vi "Create Sysdef Channels from DMAs Configuration.vi"(6 "Use NI-VS":bool, 8 "error in (no error)":errorcluster, 10 "Device Ref":T1=18446744073709551615 format="%.0x", 11 "DMAs":T2[](array[typedef])) -> (0 "error out":errorcluster, 3 "Device Ref Out":T1=18446744073709551615 format="%.0x")   [LabVIEW 2019, in "RefMem DMA System Explorer.lvlib"]
uses:
  controls/Typedef_DMA Instance.ctl
  controls/Typedef_DMA Block Settings.ctl
  controls/Data Channel Type.ctl
  controls/Typedef_Channel Settings.ctl
  <vilib>/NI VeriStand/Custom Device API/Custom Device Item Ref.ctl
  <vilib>/NI VeriStand/Custom Device API/Custom Device Channel.ctl
  <vilib>/NI VeriStand/Custom Device API/Custom Device Channel Type.ctl
  Shared/Constants.vi
  <vilib>/NI VeriStand/Custom Device API/Set Item Property (U16).vi
  <vilib>/NI VeriStand/Custom Device API/Set Item Property (U32).vi
  RefMem DMA System Explorer.lvlib
  <vilib>/NI VeriStand/Custom Device API/Custom Device API.lvlib
  Shared/RefMem DMA Shared.lvlib
panel:
  out "Creation Progress":u32(slide) scale=0.0..100.0
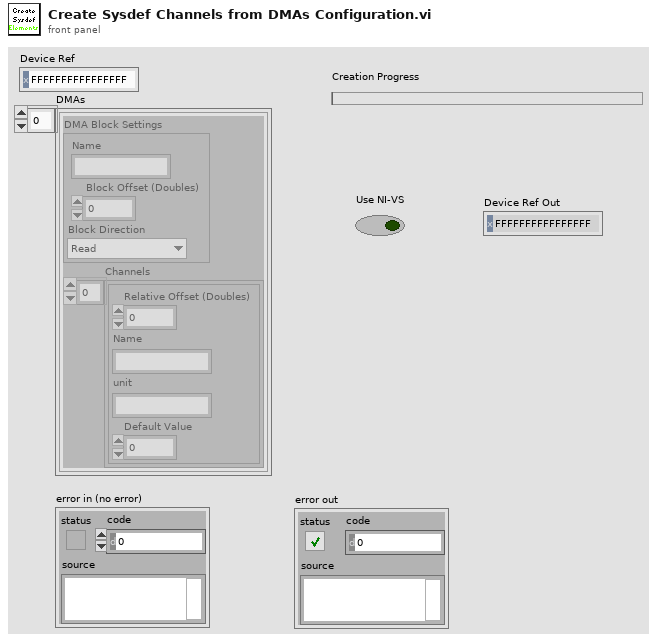
[diagram p1: front panel]
types:
  T1 = typedef "Custom Device API.lvlib/Custom Device Item Ref.ctl" = u64
  T2 = typedef "RefMem DMA System Explorer.lvlib/Typedef_DMA Instance.ctl" = cluster{"DMA Block Settings":T3, "Channels":T5[]}
  T3 = typedef "RefMem DMA System Explorer.lvlib/Typedef_DMA Block Settings.ctl" = cluster{"Name":string, " Block Offset (Doubles)":u32, "Block Direction":T4}
  T4 = typedef "RefMem DMA System Explorer.lvlib/Data Channel Type.ctl" = enum16{"Read", "Write"}
  T5 = typedef "RefMem DMA System Explorer.lvlib/Typedef_Channel Settings.ctl" = cluster{"Relative Offset (Doubles)":u32, "Name":string, "unit":string, "Default Value":dbl}
  T6 = typedef "Custom Device API.lvlib/Custom Device Channel.ctl" = cluster{"Type":T7, "Units":string, "Default Value":dbl, "Faultable":bool, "Scalable":bool}
  T7 = typedef "Custom Device API.lvlib/Custom Device Channel Type.ctl" = enum16{"Input", "Output"}
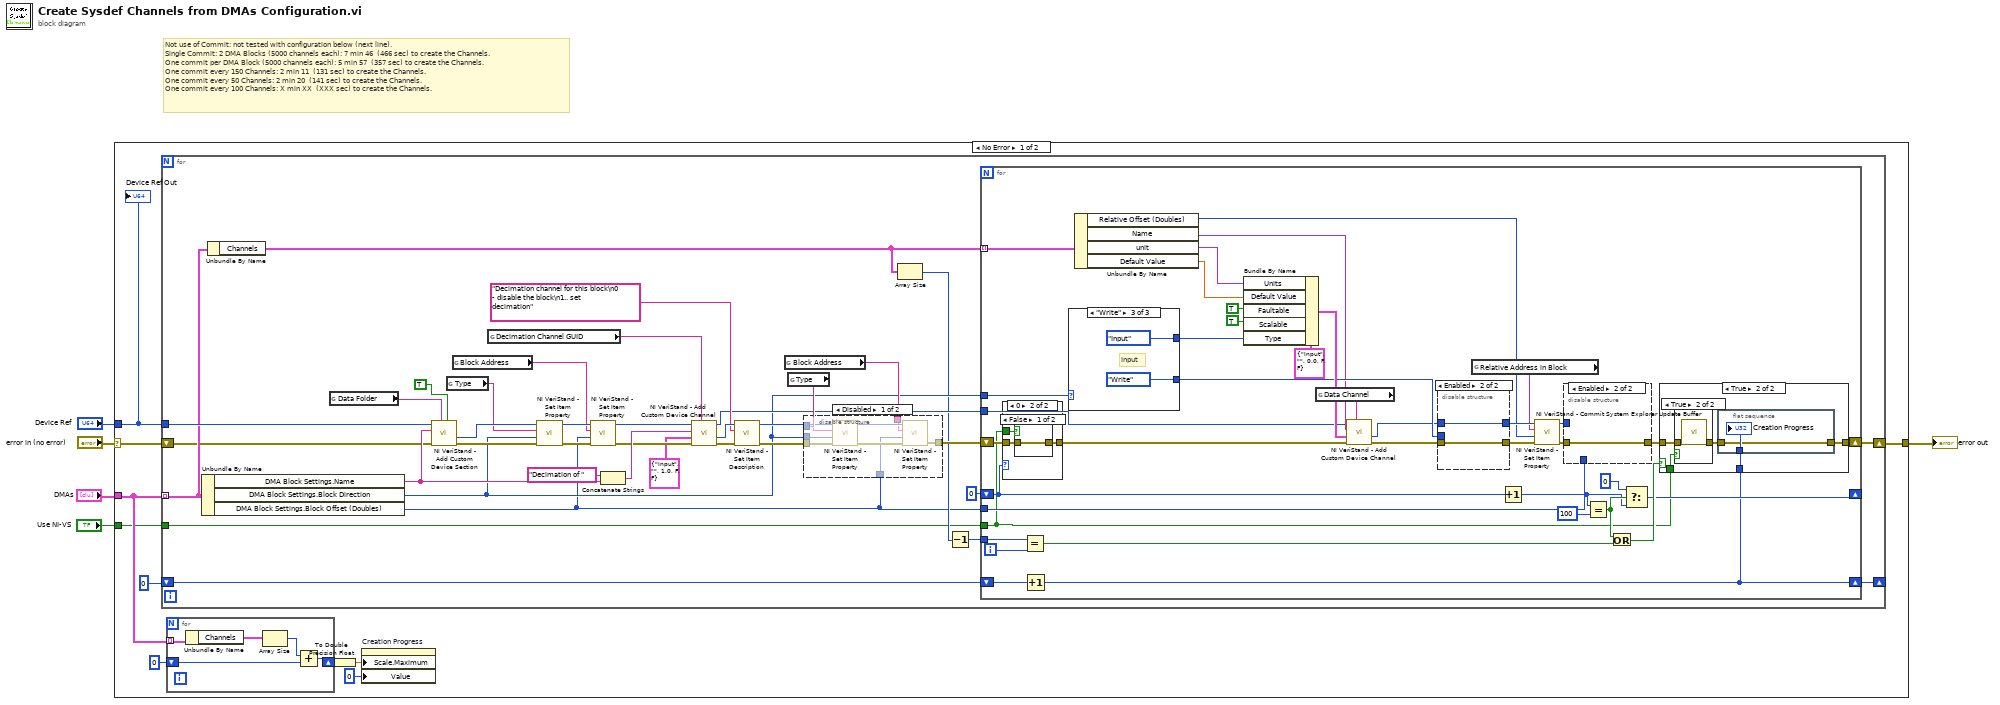
[diagram p0: block diagram]
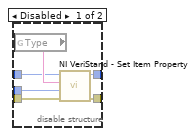
[diagram p3: hidden frame]
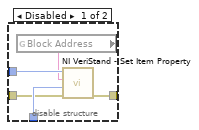
[diagram p4: hidden frame]
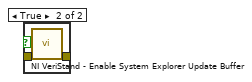
[diagram p6: hidden frame]
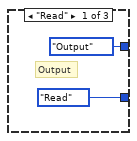
[diagram p9: hidden frame]
diagram:
  # "Not use of Commit: not tested with configuration below (next line).\nSingle Commit: 2 DMA Blocks (5000 channels each): 7 min 46  (466 sec) to create the Channels.\nOne commit per DMA Block (5000 channels each): 5 min 57  (357 sec) to create the Channels.\nOne commit every 150 Channels: 2 min 11  (131 sec) to create the Channels.\nOne commit every 50 Channels: 2 min 20  (141 sec) to create the Channels.\nOne commit every 100 Channels: X min XX  (XXX sec) to create the Channels."
  n1 = case shown="No Error" "error in (no error)" {
    selector: "error in (no error)" -> [w7 w143]
    tunnel: "Device Ref" -> [w15 _]
    tunnel: [w14 w143] -> w4
    tunnel: "DMAs" -> [w13 _]
    tunnel: "Use NI-VS" -> [w6 _]
    frame No Error {
      n2 = for {
        shift-right: [w29] -> w14
        shift-left: w7 -> [w30]
        tunnel: w15 -> [w36]
        tunnel: w13 -> [w34] mode=indexing
        shift-right: [w23] -> _
        shift-left: u32 0 -> [w24]
        tunnel: w6 -> [w21]
        n3 = Unbundle By Name(w34) -> ("DMA Block Settings.Name"=w37:string, "DMA Block Settings.Block Direction"=w31:T4, "DMA Block Settings.Block Offset (Doubles)"=w22:u32)
        n4 = Unbundle By Name(w34) -> ("Channels"=w28:T5[])
        n5 = global read "Constants.vi" "Data Folder"() -> (w42:string)
        n6 = call <vilib>:"NI VeriStand - Add Custom Device Section.vi"("Highlight? (F)"=TRUE, "GUID (Default Section)"=w42, "error in (no error)"=w30, "Section Name"=w37, "Parent Ref in"=w36) -> ("error out"=w45:errorcluster, "Section Ptr"=w49:T1)  [unwired: 3 in, 2 out]
        n7 = global read "Constants.vi" "Type"() -> (w44:string)
        n8 = global read "Constants.vi" "Block Address"() -> (w43:string)
        n9 = global read "Constants.vi" "Decimation Channel GUID"() -> (w52:string)
        n10 = call-poly <vilib>:"NI VeriStand - Set Item Property.vi"("error in (no error)"=w45, "Value"=w31, "Property Name"=w44, "Item Ref in"=w49) -> ("error out"=w46:errorcluster, "Item Ref out"=w47:T1)  [unwired: 5 in, 1 out]
        n11 = call-poly <vilib>:"NI VeriStand - Set Item Property.vi"("error in (no error)"=w46, "Value"=w22, "Property Name"=w43, "Item Ref in"=w47) -> ("error out"=w48:errorcluster, "Item Ref out"=w50:T1)  [unwired: 5 in, 1 out]
        n12 = Concatenate Strings("Decimation of " ("string"), w37) -> (w51:string)
        n13 = call <vilib>:"NI VeriStand - Add Custom Device Channel.vi"("GUID (Default Channel)"=w52, "error in (no error)"=w48, "Channel"=T6 {"Type"=enum."Input", "Units"="", "Default Value"=1.0, "Faultable"=FALSE, "Scalable"=FALSE}, "Channel Name"=w51, "Parent Ref in"=w50) -> ("error out"=w53:errorcluster, "Channel Ref"=w54:T1, "Parent Ref out"=w32:T1)  [unwired: 3 in, 1 out]
        n14 = call <vilib>:"NI VeriStand - Set Item Description.vi"("error in (no error)"=w53, "Description"="Decimation channel for this block\n0 - disable the block\n1.. set decimation" ("Section Name"), "Item Ref in"=w54) -> ("error out"=w56:errorcluster, "Item Ref out"=w33:T1)  [unwired: 6 in, 1 out]
        n15 = global read "Constants.vi" "Block Address"() -> (w57:string)
        n16 = global read "Constants.vi" "Type"() -> (w55:string)
        n17 = disable-structure shown="Disabled" {
          disable-tunnel: w57 -> [w64 _]
          disable-tunnel: w56 -> [w63 w67]
          disable-tunnel: w55 -> [w62 _]
          disable-tunnel: [w61 w67] -> w35
          disable-tunnel: w22 -> [w60 _]
          disable-tunnel: w33 -> [w59 _]
          disable-tunnel: w31 -> [w58 _]
          frame Disabled {
            n18 = call-poly <vilib>:"NI VeriStand - Set Item Property.vi"("error in (no error)"=w63, "Value"=w58, "Property Name"=w62, "Item Ref in"=w59) -> ("error out"=w66:errorcluster, "Item Ref out"=w65:T1)  [unwired: 5 in, 1 out]
            n19 = call-poly <vilib>:"NI VeriStand - Set Item Property.vi"("error in (no error)"=w66, "Value"=w60, "Property Name"=w64, "Item Ref in"=w65) -> ("error out"=w61:errorcluster)  [unwired: 5 in, 2 out]
          }
          frame Enabled {
          }
        }
        n20 = Array Size(array=w28) -> (size(s)=w26:i32)
        n21 = Decrement(x=w26) -> (x-1=w25:i32)
        n22 = for {
          shift-right: [w81] -> w29
          shift-left: w35 -> [w78]
          tunnel: w22 -> [w96]
          tunnel: w28 -> [w93] mode=indexing
          tunnel: w31 -> [w94]
          tunnel: w32 -> [w85]
          shift-right: [w74] -> _
          shift-left: 0 -> [w76]
          tunnel: w25 -> [w83]
          shift-right: [w69] -> w23
          shift-left: w24 -> [w70]
          tunnel: w21 -> [w68]
          i -> [w84]
          n23 = case shown="0" w76 {
            tunnel: w78 -> [w121 w124]
            tunnel: [w121 w123] -> w77
            tunnel: w68 -> [_ w122]
            frame 1, Default {
            }
            frame 0 {
              n24 = case shown="False" w122 {
                tunnel: w124 -> [w125 w127]
                tunnel: [w125 w126] -> w123
                frame False {
                }
                frame True {
                  n25 = call <vilib>:"NI VeriStand - Enable System Explorer Update Buffer.vi"("error in (no error)"=w127) -> ("error out"=w126:errorcluster)  [unwired: 10 in]
                }
              }
            }
          }
          n26 = Equal?(x=w83, y=w84) -> (x = y?=w80:bool)
          n27 = Increment(x=w70) -> (x+1=w69:u32)
          n28 = case shown="\"Write\"" w94 {
            tunnel: [Data_Channel_Type."Read" ("Type") _ Data_Channel_Type."Write" ("Type")] -> w102
            tunnel: [Custom_Device_Channel_Type."Output" ("Type") _ Custom_Device_Channel_Type."Input" ("Type")] -> w92
            frame "Read" {
              # "Output"
            }
            frame Default {
            }
            frame "Write" {
              # "Input"
            }
          }
          n29 = Unbundle By Name(w93) -> ("Relative Offset (Doubles)"=w88:u32, "Name"=w89:string, "unit"=w90:string, "Default Value"=w91:dbl)
          n30 = Bundle By Name(cluster=T6 {"Type"=enum."Input", "Units"="", "Default Value"=0.0, "Faultable"=FALSE, "Scalable"=FALSE} ("Channel"), "Units"=w90, "Default Value"=w91, "Faultable"=TRUE, "Scalable"=TRUE, "Type"=w92) -> (w105:T6)
          n31 = global read "Constants.vi" "Data Channel"() -> (w98:string)
          n32 = call <vilib>:"NI VeriStand - Add Custom Device Channel.vi"("GUID (Default Channel)"=w98, "error in (no error)"=w77, "Channel"=w105, "Channel Name"=w89, "Parent Ref in"=w85) -> ("error out"=w87:errorcluster, "Channel Ref"=w86:T1)  [unwired: 3 in, 2 out]
          n33 = disable-structure shown="Enabled" {
            disable-tunnel: w102 -> [w112 _]
            disable-tunnel: [w111 w114] -> w101
            disable-tunnel: [w110 w113] -> w100
            disable-tunnel: w87 -> [w108 w113]
            disable-tunnel: w86 -> [w107 w114]
            frame Disabled {
              n34 = global read "Constants.vi" "Type"() -> (w109:string)
              n35 = call-poly <vilib>:"NI VeriStand - Set Item Property.vi"("error in (no error)"=w108, "Value"=w112, "Property Name"=w109, "Item Ref in"=w107) -> ("error out"=w110:errorcluster, "Item Ref out"=w111:T1)  [unwired: 5 in, 1 out]
            }
            frame Enabled {
            }
          }
          n36 = global read "Constants.vi" "Relative Address in Block"() -> (w99:string)
          n37 = Increment(x=w76) -> (x+1=w72:i32)
          n38 = call-poly <vilib>:"NI VeriStand - Set Item Property.vi"("error in (no error)"=w100, "Value"=w88, "Property Name"=w99, "Item Ref in"=w101) -> ("error out"=w95:errorcluster, "Item Ref out"=w97:T1)  [unwired: 5 in, 1 out]
          n39 = disable-structure shown="Enabled" {
            disable-tunnel: w97 -> [w119 _]
            disable-tunnel: w96 -> [w118 _]
            disable-tunnel: w95 -> [w117 w120]
            disable-tunnel: [w115 w120] -> w82
            frame Disabled {
              n40 = global read "Constants.vi" "Block Address"() -> (w116:string)
              n41 = call-poly <vilib>:"NI VeriStand - Set Item Property.vi"("error in (no error)"=w117, "Value"=w118, "Property Name"=w116, "Item Ref in"=w119) -> ("error out"=w115:errorcluster)  [unwired: 5 in, 2 out]
            }
            frame Enabled {
            }
          }
          n42 = Equal?(x=w72, y=100) -> (x = y?=w75:bool)
          n43 = Or(x=w75, y=w80) -> (x .or. y?=w79:bool)
          n44 = Select(t=0, s=w75, f=w72) -> (s? t:f=w74:i32)
          n45 = case shown="True" w79 {
            tunnel: w82 -> [w128 w133]
            tunnel: [w128 w130] -> w81
            tunnel: w69 -> [_ w131]
            tunnel: w68 -> [_ w129]
            frame False {
            }
            frame True {
              n46 = case shown="True" w129 {
                tunnel: w133 -> [w134 w136]
                tunnel: [w134 w135] -> w132
                frame False {
                }
                frame True {
                  n47 = call <vilib>:"NI VeriStand - Commit System Explorer Update Buffer.vi"("error in (no error)"=w136) -> ("error out"=w135:errorcluster)  [unwired: 10 in]
                }
              }
              n48 = flat-sequence {
                tunnel: w132 -> [w137]
                tunnel: w131 -> [w138]
                tunnel: [w137] -> w130
                frame #0 {
                  "Creation Progress" <- w138
                }
              }
            }
          }
        }
      }
      n49 = for {
        tunnel: w13 -> [w20] mode=indexing
        shift-right: [w16] -> w11
        shift-left: 0 -> [w17]
        n50 = Unbundle By Name(w20) -> ("Channels"=w19:T5[])
        n51 = Array Size(array=w19) -> (size(s)=w18:i32)
        n52 = Add(x=w18, y=w17) -> (x+y=w16:i32)
      }
      n53 = To Double Precision Float(number=w11) -> (double precision float=w10:dbl)
      n54 = property on="Creation Progress" class="Slide (strict)"("Scale.Maximum"=w10, "Value"=u32 0 ("Creation Progress")) -> ()  [unwired: 2 in, 2 out]
      "Device Ref Out" <- w15
    }
    frame Error {
    }
  }
  "error out" <- w4
